vi "APG_Query.vi"(0 "System no.":i32=1 min=1 max=4 step=1, 2 "Channel to query":string[](array[string]), 3 "All channels?":bool, 4 "Channel identifier?":bool=TRUE, 5 "error in":errorcluster) -> (14 "APG state":dbl[](array[numeric]) format="%.6f", 19 "error out":errorcluster)   [LabVIEW 2020]
doc: "Returns Auto Piezo Gain calibration state for specified Nexline Channels.\n\nE-755: If All channels? = TRUE, then Channel identifier? must be FALSE. Command not available for E-755.101."
panel:
  # "Returns Auto Piezo Gain calibration state for specified Nexline Channels."
  # "If all channels: use"
  # "Query"
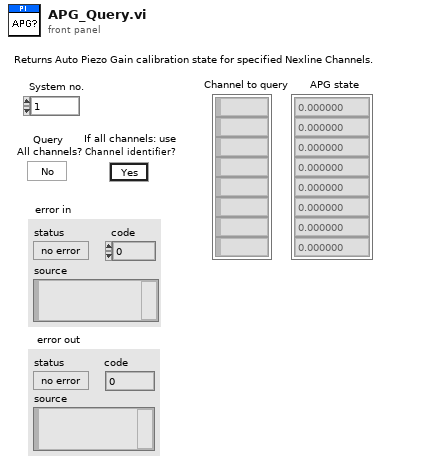
[diagram p1: front panel]
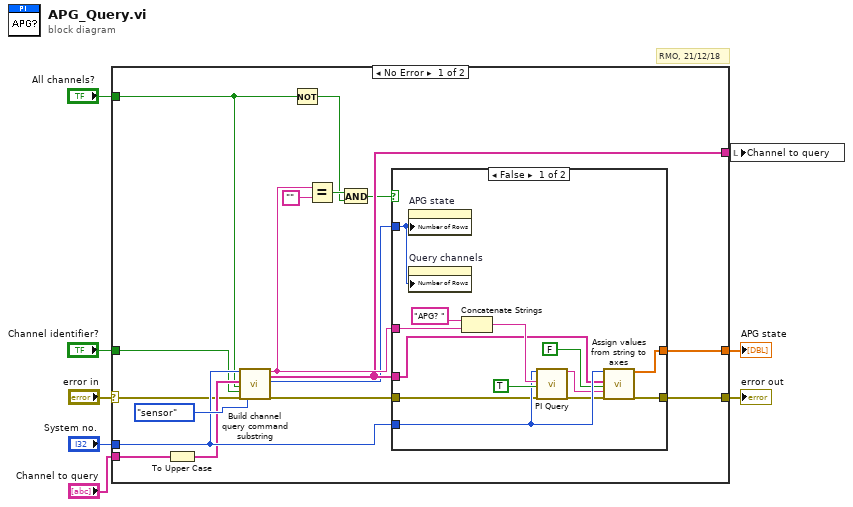
[diagram p0: block diagram]
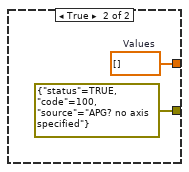
[diagram p2: hidden frame]
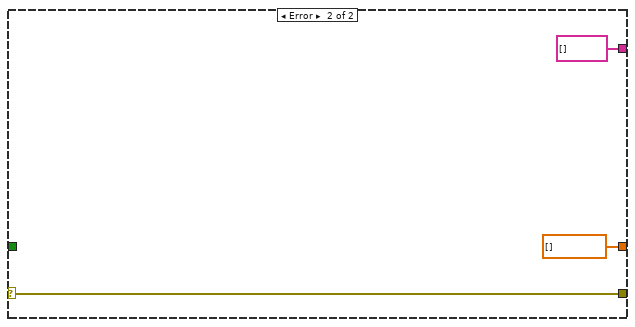
[diagram p3: hidden frame]
diagram:
  # "RMO, 21/12/18"
  n1 = case shown="No Error" "error in" {
    selector: "error in" -> [w11 w41]
    tunnel: [w25 dbl[] [] ("Values")] -> w8
    tunnel: "Channel to query" -> [w24 _]
    tunnel: [w10 w41] -> w6
    tunnel: "Channel identifier?" -> [w14 _]
    tunnel: "System no." -> [w19 _]
    tunnel: [w13 string[] [] ("Axes to query out")] -> w3
    tunnel: "All channels?" -> [w15 _]
    frame No Error {
      n2 = To Upper Case(1:w24) -> (0:w16:string[])
      n3 = call "Build channel query command substring.vi"("System no."=w19, "Channels to query in"=w16, "Query\nAll channels?"=w15, "For all channels: use\nChannel identifier?"=w14, "error in"=w11, "Channel type"=enum16{"piezo", "sensor"}."sensor") -> ("Command substring"=w18:string, "Channels to query out"=w13:string[], "Number of rows"=w12:u32, "error out"=w17:errorcluster)  [unwired: 1 in, 9 out]
      n4 = Not(x=w15) -> (.not. x?=w21:bool)
      n5 = Equal?(x=w18, y="" ("x")) -> (x = y?=w22:bool)
      n6 = And(x=w22, y=w21) -> (x .and. y?=w9:bool)
      n7 = case shown="False" w9 {
        tunnel: [w35 w39] -> w25
        tunnel: w19 -> [w34 _]
        tunnel: w18 -> [w33 _]
        tunnel: w17 -> [w32 _]
        tunnel: w13 -> [w31 _]
        tunnel: w12 -> [w30 _]
        tunnel: [w28 errorcluster {"status"=TRUE, "code"=100, "source"="APG? no axis specified"} ("error out")] -> w10
        frame False {
          n8 = property on="APG state" class="Arr (strict)"("Number of Rows"=w30) -> ()  [unwired: 2 in, 2 out]
          n9 = property on="Query channels" class="Arr (strict)"("Number of Rows"=w30) -> ()  [unwired: 2 in, 2 out]
          n10 = Concatenate Strings("APG? ", w33) -> (w36:string)
          n11 = call "PI Query.vi"("System no."=w34, "String to send"=w36, "Attach termination char.?"=TRUE ("Attach Linefeed?"), "error in"=w32) -> ("String read"=w26:string, "error out"=w27:errorcluster)  [unwired: 3 in, 11 out]
          n12 = call "Assign values from string to axes.vi"("System no."=w34, "Queried axes"=w31, "All axes queried?"=FALSE, "Input String"=w26, "error in"=w27) -> ("Values"=w35:dbl[], "error out"=w28:errorcluster)  [unwired: 4 in, 9 out]
        }
        frame True {
          w39 = dbl[] []  # Values
        }
      }
    }
    frame Error {
    }
  }
  "error out" <- w6
  "APG state" <- w8
  n13 = local write "Channel to query"(w3) -> ()
